vi "New Heartbeat Message.vi"() -> (0 "Heartbeat Message":T1={"type"="heartbeat", "message"="{}"})   [LabVIEW 2016]
uses:
  Heartbeat Message.ctl
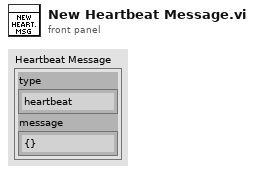
[diagram p1: front panel]
types:
  T1 = typedef "Heartbeat Message.ctl" = cluster{"type":string, "message":string}
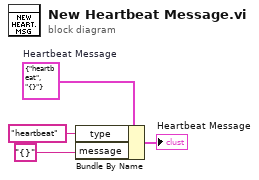
[diagram p0: block diagram]
diagram:
  w2 = T1 {"type"="heartbeat", "message"="{}"}  # Heartbeat Message
  n1 = Bundle By Name(cluster=w2, "type"="heartbeat" ("Type"), "message"="{}" ("Message")) -> (→"Heartbeat Message":T1)
